vi "TempAlgoTest (SubVI).vi"(0 "Temp":refnum<vi>, 1 "Speed Ind":dbl format="%#_13g", 2 "Motor Speed RPM":refnum<vi>, 3 "Round":T1(ring), 4 "Temp Up In":dbl format="%#_13g", 5 "error in (no error)":errorcluster, 6 "String in":refnum<vi>, 7 "Temp Goal":dbl format="%#_13g", 8 "Stop":refnum<vi>, 9 "Speed Goal":dbl format="%#_13g", 10 "Stop BurnIn":refnum<vi>, 11 "AD Resistor Step":dbl=9.0 format="%#_13g", 12 "Strin":string) -> (14 "Speed Pass/Fail":bool, 15 "Temp  Pass/Fail":dbl, 16 "Temp Up Out":dbl, 17 "Speed Pass/Fail":dbl, 18 "Temp Pass/Fail":bool, 19 "error out":errorcluster)   [LabVIEW 2017]
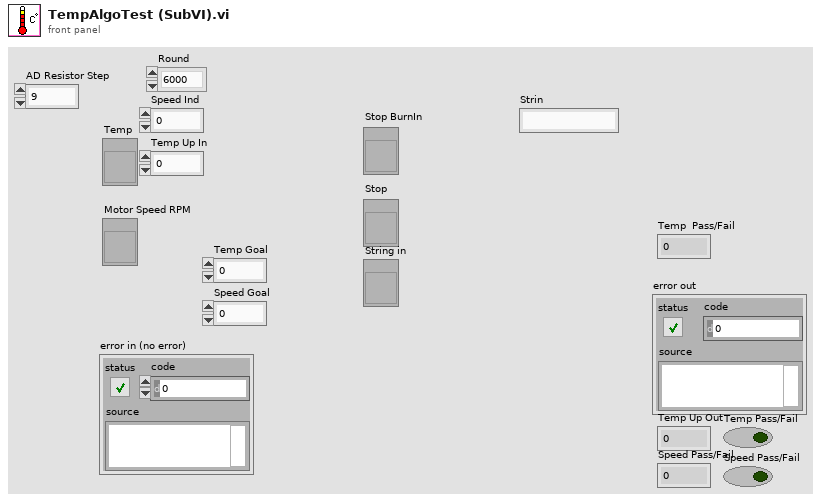
[diagram p1: front panel]
types:
  T1 = enum32{"6000", "11500", "15100", "11500-2", "6000-2"}
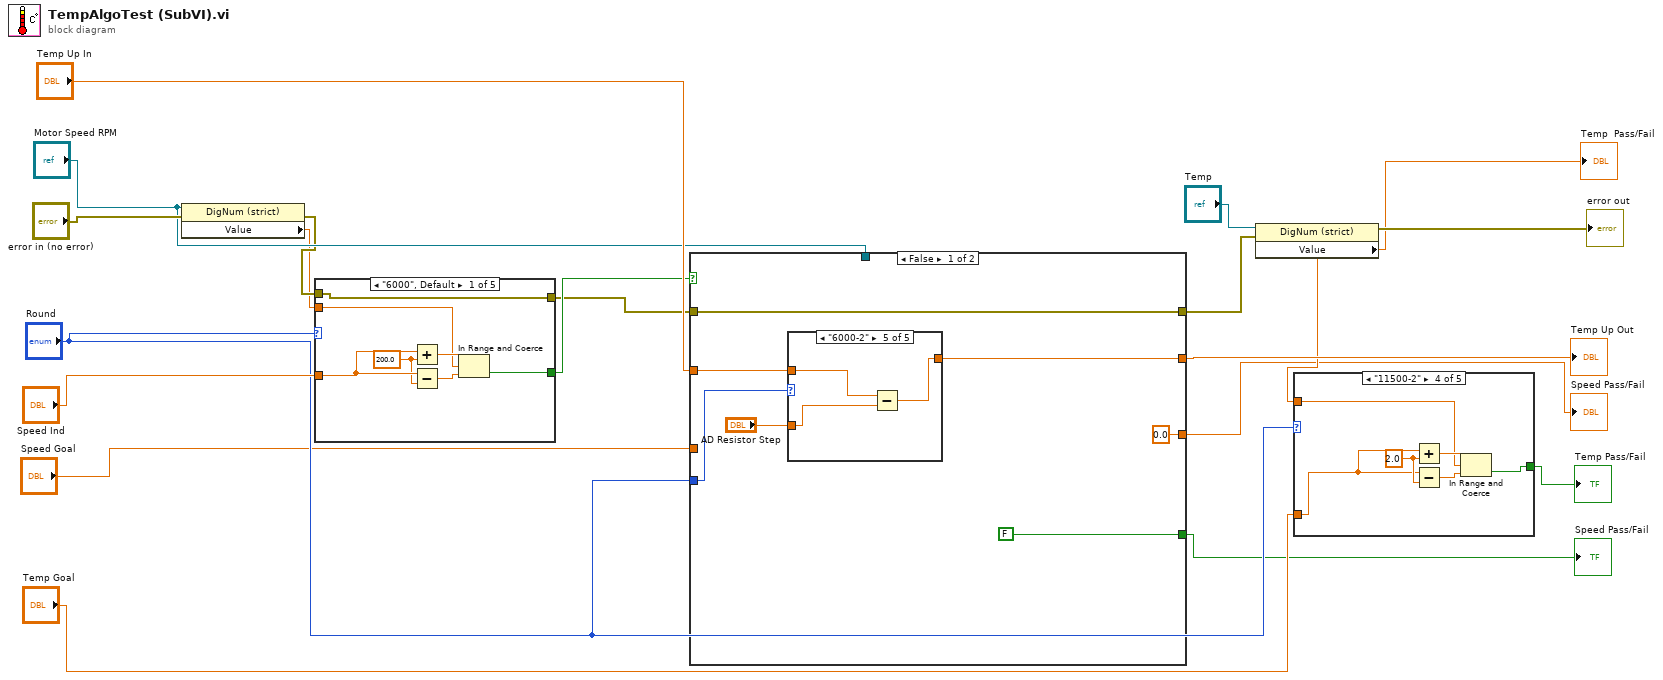
[diagram p0: block diagram]
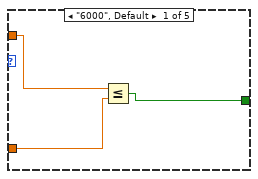
[diagram p2: hidden frame]
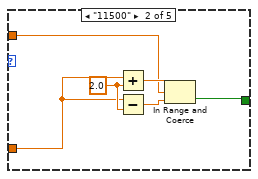
[diagram p3: hidden frame]
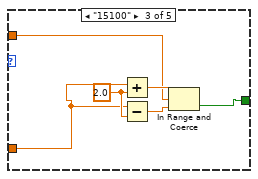
[diagram p4: hidden frame]
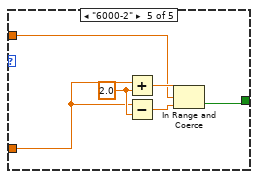
[diagram p5: hidden frame]
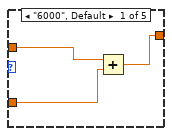
[diagram p6: hidden frame]
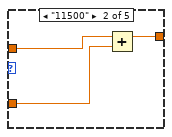
[diagram p7: hidden frame]
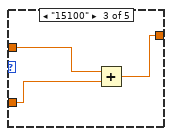
[diagram p8: hidden frame]
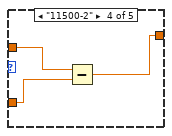
[diagram p9: hidden frame]
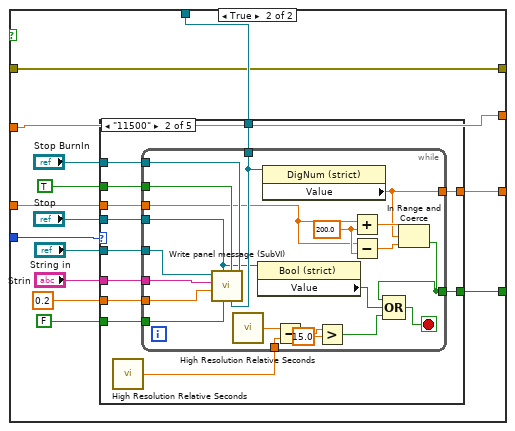
[diagram p10: hidden frame]
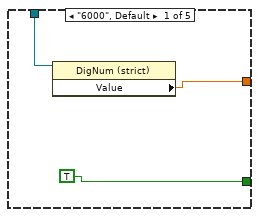
[diagram p11: hidden frame]
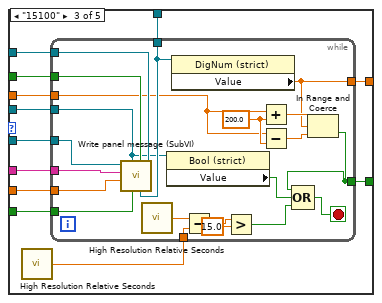
[diagram p12: hidden frame]
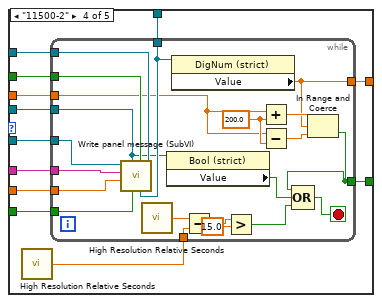
[diagram p13: hidden frame]
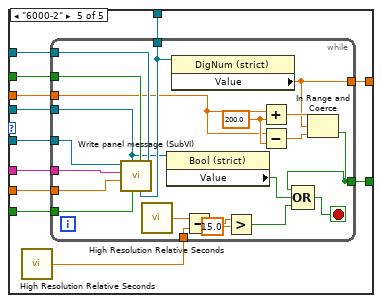
[diagram p14: hidden frame]
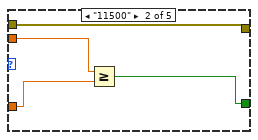
[diagram p15: hidden frame]
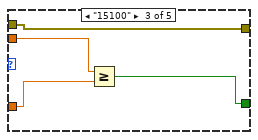
[diagram p16: hidden frame]
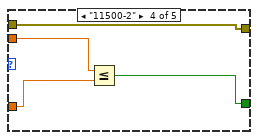
[diagram p17: hidden frame]
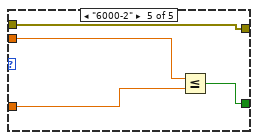
[diagram p18: hidden frame]
diagram:
  n1 = property class="DigNum (strict)"(reference="Motor Speed RPM", error in="error in (no error)") -> (error out=w6:errorcluster, "Value"=w3:dbl)  [unwired: 1 out]
  n2 = case shown="\"6000\", Default" "Round" {
    tunnel: w3 -> [w23 w30 w34 w38 w42]
    tunnel: "Speed Ind" -> [w24 w29 w33 w37 w41]
    tunnel: [w21 w28 w32 w36 w40] -> w14
    tunnel: w6 -> [w20 w27 w31 w35 w39]
    tunnel: [w20 w27 w31 w35 w39] -> w5
    frame "6000", Default {
      w22 = 200.0 ("y")
      n3 = Add(x=w24, y=w22) -> (x+y=w26:dbl)
      n4 = Subtract(x=w24, y=w22) -> (x-y=w25:dbl)
      n5 = In Range and Coerce(upper limit=w26, x=w23, lower limit=w25) -> (In Range?=w21:bool)  [unwired: 1 out]
    }
    frame "11500" {
      n6 = Greater Or Equal?(x=w30, y=w29) -> (x >= y?=w28:bool)
    }
    frame "15100" {
      n7 = Greater Or Equal?(x=w34, y=w33) -> (x >= y?=w32:bool)
    }
    frame "11500-2" {
      n8 = Less Or Equal?(x=w38, y=w37) -> (x <= y?=w36:bool)
    }
    frame "6000-2" {
      n9 = Less Or Equal?(x=w42, y=w41) -> (x <= y?=w40:bool)
    }
  }
  n10 = case shown="False" w14 {
    tunnel: "Temp Up In" -> [w49 w78]
    tunnel: [w48 w78] -> w13
    tunnel: "Motor Speed RPM" -> [_ w70]
    tunnel: "Round" -> [w44 w69]
    tunnel: [FALSE ("rpm 2") w68] -> w7
    tunnel: w5 -> [w46 w67]
    tunnel: [w46 w67] -> w4
    tunnel: "Speed Goal" -> [_ w66]
    tunnel: [0.0 ("Value") w65] -> w1
    frame False {
      n11 = case shown="\"6000-2\"" w44 {
        tunnel: w49 -> [w52 w55 w58 w61 w64]
        tunnel: [w51 w54 w57 w60 w63] -> w48
        tunnel: "AD Resistor Step" -> [w50 w53 w56 w59 w62]
        frame "6000", Default {
          n12 = Add(x=w52, y=w50) -> (x+y=w51:dbl)
        }
        frame "11500" {
          n13 = Add(x=w55, y=w53) -> (x+y=w54:dbl)
        }
        frame "15100" {
          n14 = Add(x=w58, y=w56) -> (x+y=w57:dbl)
        }
        frame "11500-2" {
          n15 = Subtract(x=w61, y=w59) -> (x-y=w60:dbl)
        }
        frame "6000-2" {
          n16 = Subtract(x=w64, y=w62) -> (x-y=w63:dbl)
        }
      }
    }
    frame True {
      n17 = case shown="\"11500\"" w69 {
        tunnel: "Stop BurnIn" -> [_ w93 w126 w159 w192]
        tunnel: TRUE ("rpm 2") -> [_ w92 w125 w158 w191]
        tunnel: FALSE ("PrintTime") -> [_ w91 w124 w157 w190]
        tunnel: "Stop" -> [_ w90 w123 w156 w189]
        tunnel: 0.2 ("Time to wait") -> [_ w89 w122 w155 w188]
        tunnel: "Strin" -> [_ w88 w121 w154 w187]
        tunnel: "String in" -> [_ w87 w120 w153 w186]
        tunnel: w70 -> [w80 w86 w119 w152 w185]
        tunnel: [TRUE ("rpm 2") w83 w116 w149 w182] -> w68
        tunnel: w66 -> [_ w85 w118 w151 w184]
        tunnel: [w79 w84 w117 w150 w183] -> w65
        frame "6000", Default {
          n18 = property class="DigNum (strict)"(reference=w80) -> ("Value"=w79:dbl)  [unwired: 1 in, 2 out]
        }
        frame "11500" {
          n19 = call <vilib>:"High Resolution Relative Seconds.vi"() -> ("relative seconds"=w82:dbl)
          n20 = while {
            tunnel: w93 -> [w114]
            tunnel: w92 -> [w113]
            tunnel: w91 -> [w112]
            tunnel: w90 -> [w107]
            tunnel: w89 -> [w111]
            tunnel: w88 -> [w110]
            tunnel: w87 -> [w109]
            tunnel: w86 -> [w108]
            tunnel: w85 -> [w103]
            tunnel: [w102] -> w84
            tunnel: [w100] -> w83
            tunnel: w82 -> [w97]
            stop <- w101 stop-if-true
            w106 = 200.0 ("y")
            n21 = call "Write panel message (SubVI).vi"("Stop BurnIn"=w114, 4:"rpm"=w108, 5:"rpm"=w113, "PrintTime"=w112, "Stop"=w107, "Time to wait"=w111, "Strin"=w110, "String in"=w109) -> ()  [unwired: 3 in, 1 out]
            n22 = call <vilib>:"High Resolution Relative Seconds.vi"() -> ("relative seconds"=w98:dbl)
            n23 = property class="Bool (strict)"(reference=w107) -> ("Value"=w99:bool)  [unwired: 1 in, 2 out]
            n24 = property class="DigNum (strict)"(reference=w108) -> ("Value"=w102:dbl)  [unwired: 1 in, 2 out]
            n25 = Subtract(x=w98, y=w97) -> (x-y=w96:dbl)
            n26 = Greater?(x=w96, y=15.0) -> (0:w94:bool)
            n27 = Add(x=w103, y=w106) -> (x+y=w104:dbl)
            n28 = Subtract(x=w103, y=w106) -> (x-y=w105:dbl)
            n29 = In Range and Coerce(upper limit=w104, x=w102, lower limit=w105) -> (In Range?=w100:bool)  [unwired: 1 out]
            n30 = Compound Arithmetic op=OR(w100, w99, w94) -> (w101:bool)
          }
        }
        frame "15100" {
          n31 = call <vilib>:"High Resolution Relative Seconds.vi"() -> ("relative seconds"=w115:dbl)
          n32 = while {
            tunnel: w126 -> [w147]
            tunnel: w125 -> [w146]
            tunnel: w124 -> [w145]
            tunnel: w123 -> [w140]
            tunnel: w122 -> [w144]
            tunnel: w121 -> [w143]
            tunnel: w120 -> [w142]
            tunnel: w119 -> [w141]
            tunnel: w118 -> [w136]
            tunnel: [w135] -> w117
            tunnel: [w133] -> w116
            tunnel: w115 -> [w130]
            stop <- w134 stop-if-true
            w139 = 200.0 ("y")
            n33 = call "Write panel message (SubVI).vi"("Stop BurnIn"=w147, 4:"rpm"=w141, 5:"rpm"=w146, "PrintTime"=w145, "Stop"=w140, "Time to wait"=w144, "Strin"=w143, "String in"=w142) -> ()  [unwired: 3 in, 1 out]
            n34 = call <vilib>:"High Resolution Relative Seconds.vi"() -> ("relative seconds"=w131:dbl)
            n35 = property class="Bool (strict)"(reference=w140) -> ("Value"=w132:bool)  [unwired: 1 in, 2 out]
            n36 = property class="DigNum (strict)"(reference=w141) -> ("Value"=w135:dbl)  [unwired: 1 in, 2 out]
            n37 = Subtract(x=w131, y=w130) -> (x-y=w129:dbl)
            n38 = Greater?(x=w129, y=15.0) -> (0:w127:bool)
            n39 = Add(x=w136, y=w139) -> (x+y=w137:dbl)
            n40 = Subtract(x=w136, y=w139) -> (x-y=w138:dbl)
            n41 = In Range and Coerce(upper limit=w137, x=w135, lower limit=w138) -> (In Range?=w133:bool)  [unwired: 1 out]
            n42 = Compound Arithmetic op=OR(w133, w132, w127) -> (w134:bool)
          }
        }
        frame "11500-2" {
          n43 = call <vilib>:"High Resolution Relative Seconds.vi"() -> ("relative seconds"=w148:dbl)
          n44 = while {
            tunnel: w159 -> [w180]
            tunnel: w158 -> [w179]
            tunnel: w157 -> [w178]
            tunnel: w156 -> [w173]
            tunnel: w155 -> [w177]
            tunnel: w154 -> [w176]
            tunnel: w153 -> [w175]
            tunnel: w152 -> [w174]
            tunnel: w151 -> [w169]
            tunnel: [w168] -> w150
            tunnel: [w166] -> w149
            tunnel: w148 -> [w163]
            stop <- w167 stop-if-true
            w172 = 200.0 ("y")
            n45 = call "Write panel message (SubVI).vi"("Stop BurnIn"=w180, 4:"rpm"=w174, 5:"rpm"=w179, "PrintTime"=w178, "Stop"=w173, "Time to wait"=w177, "Strin"=w176, "String in"=w175) -> ()  [unwired: 3 in, 1 out]
            n46 = call <vilib>:"High Resolution Relative Seconds.vi"() -> ("relative seconds"=w164:dbl)
            n47 = property class="Bool (strict)"(reference=w173) -> ("Value"=w165:bool)  [unwired: 1 in, 2 out]
            n48 = property class="DigNum (strict)"(reference=w174) -> ("Value"=w168:dbl)  [unwired: 1 in, 2 out]
            n49 = Subtract(x=w164, y=w163) -> (x-y=w162:dbl)
            n50 = Greater?(x=w162, y=15.0) -> (0:w160:bool)
            n51 = Add(x=w169, y=w172) -> (x+y=w170:dbl)
            n52 = Subtract(x=w169, y=w172) -> (x-y=w171:dbl)
            n53 = In Range and Coerce(upper limit=w170, x=w168, lower limit=w171) -> (In Range?=w166:bool)  [unwired: 1 out]
            n54 = Compound Arithmetic op=OR(w166, w165, w160) -> (w167:bool)
          }
        }
        frame "6000-2" {
          n55 = call <vilib>:"High Resolution Relative Seconds.vi"() -> ("relative seconds"=w181:dbl)
          n56 = while {
            tunnel: w192 -> [w213]
            tunnel: w191 -> [w212]
            tunnel: w190 -> [w211]
            tunnel: w189 -> [w206]
            tunnel: w188 -> [w210]
            tunnel: w187 -> [w209]
            tunnel: w186 -> [w208]
            tunnel: w185 -> [w207]
            tunnel: w184 -> [w202]
            tunnel: [w201] -> w183
            tunnel: [w199] -> w182
            tunnel: w181 -> [w196]
            stop <- w200 stop-if-true
            w205 = 200.0 ("y")
            n57 = call "Write panel message (SubVI).vi"("Stop BurnIn"=w213, 4:"rpm"=w207, 5:"rpm"=w212, "PrintTime"=w211, "Stop"=w206, "Time to wait"=w210, "Strin"=w209, "String in"=w208) -> ()  [unwired: 3 in, 1 out]
            n58 = call <vilib>:"High Resolution Relative Seconds.vi"() -> ("relative seconds"=w197:dbl)
            n59 = property class="Bool (strict)"(reference=w206) -> ("Value"=w198:bool)  [unwired: 1 in, 2 out]
            n60 = property class="DigNum (strict)"(reference=w207) -> ("Value"=w201:dbl)  [unwired: 1 in, 2 out]
            n61 = Subtract(x=w197, y=w196) -> (x-y=w195:dbl)
            n62 = Greater?(x=w195, y=15.0) -> (0:w193:bool)
            n63 = Add(x=w202, y=w205) -> (x+y=w203:dbl)
            n64 = Subtract(x=w202, y=w205) -> (x-y=w204:dbl)
            n65 = In Range and Coerce(upper limit=w203, x=w201, lower limit=w204) -> (In Range?=w199:bool)  [unwired: 1 out]
            n66 = Compound Arithmetic op=OR(w199, w198, w193) -> (w200:bool)
          }
        }
      }
    }
  }
  "Temp Up Out" <- w13
  "Speed Pass/Fail" <- w7
  "Speed Pass/Fail" <- w1
  n67 = property class="DigNum (strict)"(reference="Temp", error in=w4) -> (error out=→"error out":errorcluster, "Value"=w12:dbl)  [unwired: 1 out]
  "Temp  Pass/Fail" <- w12
  n68 = case shown="\"11500-2\"" "Round" {
    tunnel: w12 -> [w215 w219 w225 w231 w237]
    tunnel: [w216 w217 w223 w229 w235] -> w10
    tunnel: "Temp Goal" -> [w214 w218 w224 w230 w236]
    frame "6000", Default {
      n69 = Less Or Equal?(x=w215, y=w214) -> (x <= y?=w216:bool)
    }
    frame "11500" {
      w220 = 2.0 ("y")
      n70 = Add(x=w218, y=w220) -> (x+y=w222:dbl)
      n71 = Subtract(x=w218, y=w220) -> (x-y=w221:dbl)
      n72 = In Range and Coerce(upper limit=w222, x=w219, lower limit=w221) -> (In Range?=w217:bool)  [unwired: 1 out]
    }
    frame "15100" {
      w226 = 2.0 ("y")
      n73 = Add(x=w224, y=w226) -> (x+y=w228:dbl)
      n74 = Subtract(x=w224, y=w226) -> (x-y=w227:dbl)
      n75 = In Range and Coerce(upper limit=w228, x=w225, lower limit=w227) -> (In Range?=w223:bool)  [unwired: 1 out]
    }
    frame "11500-2" {
      w232 = 2.0 ("y")
      n76 = Add(x=w230, y=w232) -> (x+y=w234:dbl)
      n77 = Subtract(x=w230, y=w232) -> (x-y=w233:dbl)
      n78 = In Range and Coerce(upper limit=w234, x=w231, lower limit=w233) -> (In Range?=w229:bool)  [unwired: 1 out]
    }
    frame "6000-2" {
      w238 = 2.0 ("y")
      n79 = Add(x=w236, y=w238) -> (x+y=w240:dbl)
      n80 = Subtract(x=w236, y=w238) -> (x-y=w239:dbl)
      n81 = In Range and Coerce(upper limit=w240, x=w237, lower limit=w239) -> (In Range?=w235:bool)  [unwired: 1 out]
    }
  }
  "Temp Pass/Fail" <- w10
